vi "WSVCAP SHL Host LL Get Boolean Parameter.vi"(11 "error in (no error)":errorcluster, 13 "FPGA Top Level Control":T1=enum."Bytes to Write") -> (4 "Boolean Out":bool, 15 "error out":errorcluster)   [LabVIEW 2012]
uses:
  Type Defs/WSVCAP SHL Top Level Control Enum.ctl
  Type Defs/WSVCAP SHL Top Level Control Operation Enum.ctl
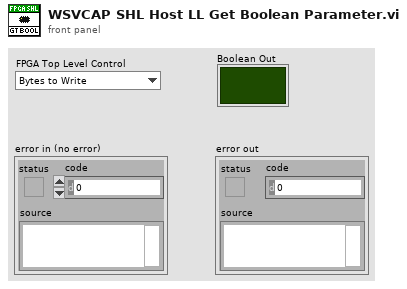
[diagram p1: front panel]
types:
  T1 = typedef "WSVCAP SHL Top Level Control Enum.ctl" = enum16{"Start", "Cmd", "Transaction", "Wait Ticks", "Socket Mask", "Slave Address", "Sub Address", "Bytes to Write", "Bytes to Read", "Write Data", "Write Flag", "Read Data", "Read Flag", "Ack Read", "Read Status Flag", "Ack Read Status", "Status", "Cycle Count", "Stop Cycle", "Exit"}
  T2 = typedef "WSVCAP SHL Top Level Control Operation Enum.ctl" = enum16{"Initialize", "Set Control", "Read Control", "Close"}
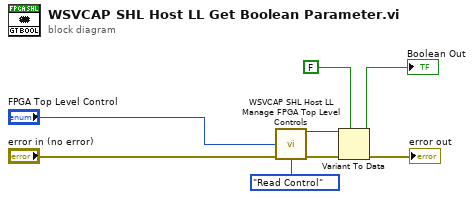
[diagram p0: block diagram]
diagram:
  n1 = call "WSVCAP SHL Host LL Manage FPGA Top Level Controls.vi"("FPGA Top Level Control"="FPGA Top Level Control", "error in (no error)"="error in (no error)", "Operation"=WSVCAP_SHL_Top_Level_Control_Operation_Enum."Read Control") -> ("Value Out"=w2:variant, "error out"=w5:errorcluster)  [unwired: 11 in]
  n2 = Variant To Data(error in=w5, type=FALSE ("Boolean"), Variant=w2) -> (data=→"Boolean Out":bool, error out=→"error out":errorcluster)
